vi "AskForImg.vi"() -> ()   [LabVIEW 2018]
uses:
  <vilib>/Instr/_visa.llb/VISA Configure Serial Port (Instr).vi
panel:
  in  "pattern":u8
  in  "chip":u8
  in  "stop":bool
  out "read buffer":string
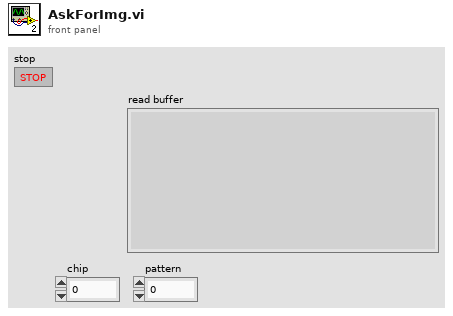
[diagram p1: front panel]
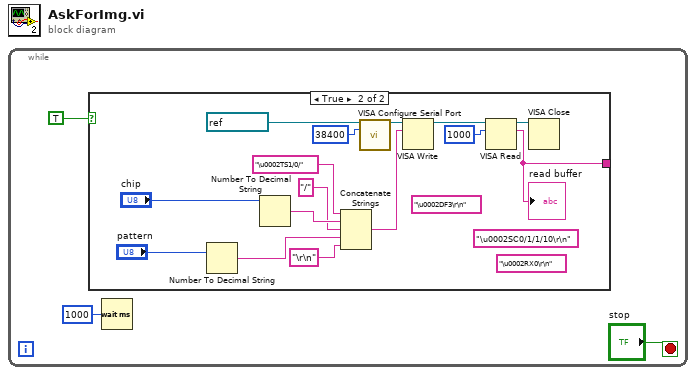
[diagram p0: block diagram]
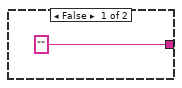
[diagram p2: hidden frame]
diagram:
  n1 = while {
    stop <- "stop" stop-if-true
    n2 = case shown="True" TRUE {
      tunnel: ["" ("read buffer") w13] -> _
      frame False {
      }
      frame True {
        (unwired) "\u0002DF3\r\n" ("format string")
        (unwired) "\u0002SC0/1/1/10\r\n" ("format string")
        (unwired) "\u0002RX0\r\n" ("format string")
        n3 = Number To Decimal String(number="pattern") -> (decimal integer string=w7:string)  [unwired: 1 in]
        n4 = Number To Decimal String(number="chip") -> (decimal integer string=w9:string)  [unwired: 1 in]
        n5 = Concatenate Strings("\u0002TS1/0/" ("format string"), w9, "/" ("string"), w7, "\r\n" ("format string")) -> (w5:string)
        n6 = call-poly "VISA Configure Serial Port"("VISA resource name"=refnum<visa-resource-name> "COM4", "baud rate (9600)"=u32 38400) -> ("VISA resource name out"=w17:refnum<visa-resource-name>)  [unwired: 12 in, 1 out]
        n7 = VISA Write(VISA resource name=w17, write buffer=w5) -> (VISA resource name out=w16:refnum<visa-resource-name>)  [unwired: 1 in, 2 out]
        n8 = VISA Read(VISA resource name=w16, byte count=u32 1000) -> (VISA resource name out=w15:refnum<visa-resource-name>, read buffer=w13:string)  [unwired: 1 in, 2 out]
        "read buffer" <- w13
        n9 = VISA Close(VISA resource name=w15) -> ()  [unwired: 1 in, 1 out]
      }
    }
    n10 = Wait (ms)(milliseconds to wait=u32 1000) -> ()  [unwired: 1 out]
  }
